vi "z maximum.vi"(8 "Error In":errorcluster, 10 "Maximum settings":T1 {"z maximum position" min=-5.0 max=105.0}, 11 "Action":T2) -> (0 "Error out":errorcluster, 2 "Z-Maximum Out":T1 {"z maximum position" min=-5.0 max=105.0})   [LabVIEW 2011]
doc: "Functional Global Variable for the algorithm settings. The used method as well as the max. Iteration steps and the tolerance can be given. In addition, the algorithm can be told to use boundaries (if possible)."
uses:
  Studium/Multilayer University of Bern Folder/controls/FGV_Action.ctl
  controls/z maximum information.ctl
panel:
  # "Input"
  # "Output"
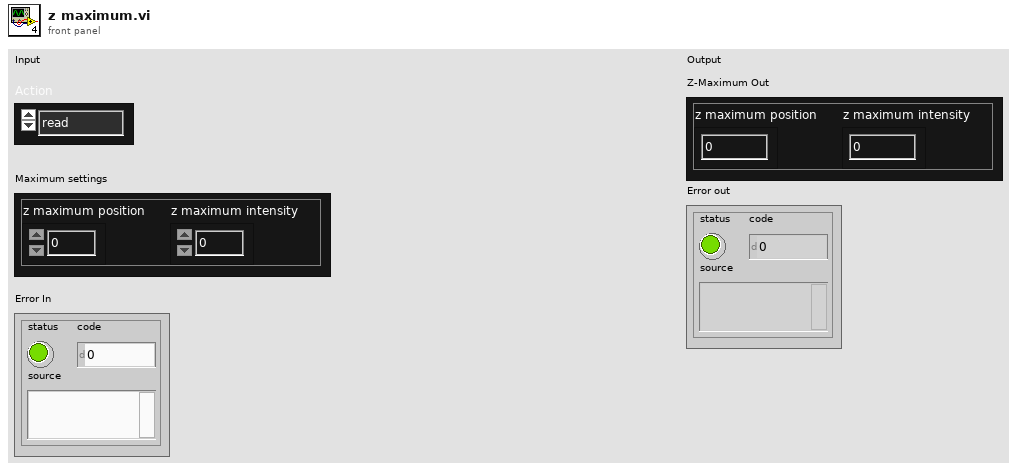
[diagram p1: front panel]
types:
  T1 = typedef "z maximum information.ctl" = cluster{"z maximum position":dbl, "z maximum intensity":dbl}
  T2 = typedef "FGV_Action.ctl" = enum16{"read", "write"}
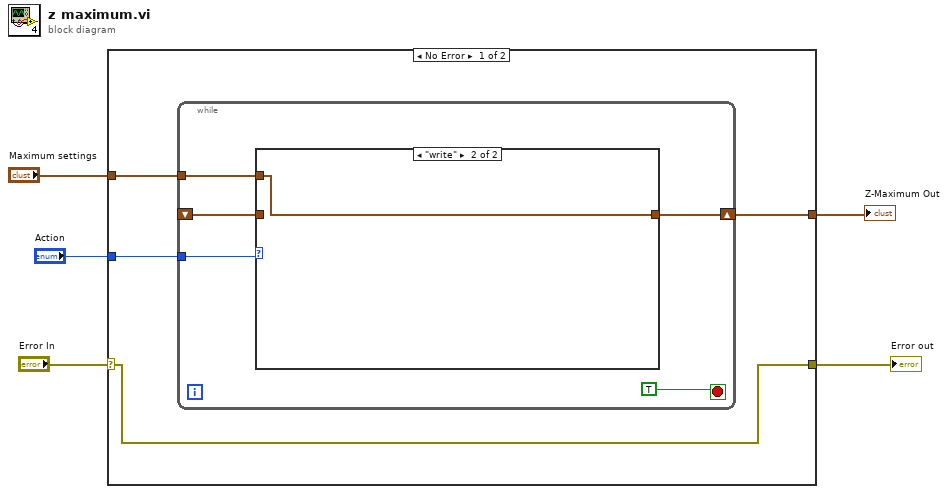
[diagram p0: block diagram]
diagram:
  n1 = case shown="No Error" "Error In" {
    selector: "Error In" -> [w6 w18]
    tunnel: "Action" -> [w9 _]
    tunnel: [w6 w18] -> w3
    tunnel: "Maximum settings" -> [w8 w17]
    tunnel: [w7 w17] -> w1
    frame No Error {
      n2 = while {
        tunnel: w9 -> [w13]
        tunnel: w8 -> [w12]
        shift-right: [w10] -> w7
        shift-left: _ -> [w11]
        stop <- TRUE stop-if-true
        n3 = case shown="\"write\"" w13 {
          tunnel: w12 -> [_ w16]
          tunnel: w11 -> [w15 _]
          tunnel: [w15 w16] -> w10
          frame "read", Default {
          }
          frame "write" {
          }
        }
      }
    }
    frame Error {
    }
  }
  "Error out" <- w3
  "Z-Maximum Out" <- w1
